vi "quotient-remainder.vi"() -> ()   [LabVIEW 2025]
panel:
  out "rem":dbl
  out "iq":dbl
  in  "b":dbl
  in  "a":dbl
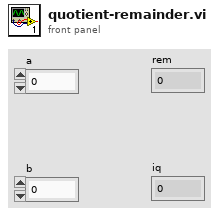
[diagram p1: front panel]
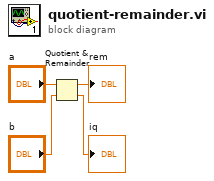
[diagram p0: block diagram]
diagram:
  n1 = Quotient & Remainder(x="a", y="b") -> (x-y*floor(x/y)=→"rem":dbl, floor(x/y)=→"iq":dbl)
